vi "prepAO_img.vi"() -> (0 "Terminal Name with Device Prefix":tag)   [LabVIEW 2015]
uses:
  <vilib>/DAQmx/write.llb/DAQmx Write (Analog 1D Wfm NChan NSamp).vi
  waveforms/usedAOindepofwf.vi
  Misc/add channel to active arrayv2.vi
  Objects/waveformsAObuffer.vi
  <vilib>/DAQmx/create/channels.llb/DAQmx Create Channel (AO-Voltage-Basic).vi
  <vilib>/DAQmx/configure/timing.llb/DAQmx Timing (Sample Clock).vi
  <vilib>/DAQmx/miscellaneous.llb/DAQmx Fill In Error Info.vi
  <vilib>/DAQmx/configure/trigger.llb/DAQmx Start Trigger (Digital Edge).vi
panel:
  in  "error in 3":errorcluster caption="error in"
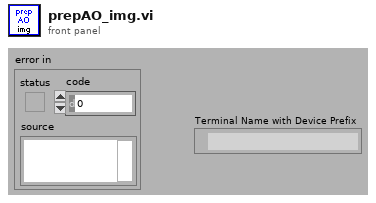
[diagram p1: front panel]
types:
  T1 = cluster{"presorted indices":i32[], "AOchans in this device":tag[], "usedAO sorted":i32[]}[]
  T2 = typedef "LVRectTypeDef.ctl" = cluster{"Left":i16, "Top":i16, "Right":i16, "Bottom":i16}
  T3 = cluster{"Xpixels":i32, "Vxminref":dbl, "Vxmaxref":dbl, "P":dbl, "Ypixels":i32, "Vyminref":dbl, "Vymaxref":dbl, "srate":sgl, "sAOxy":i32, "timeout":dbl, "type":string, "date":string, "time":string, "Colormap":u16, "Drawing Mode":u16, "Scanning Mode":u16, "square pixels":bool, "square matrix":bool, "Xpixels Img":i32, "Vx-min Img":dbl, "VX-max Img":dbl, "Ypixels Img":i32, "Vy-min Img":dbl, "Vy-max Img ":dbl, "Angle Img":dbl, "autoshutter":bool, "finite":bool, "cont":bool, "wavdet":bool, "measpoints":i32, "avpp":i32, "bufferAO":i32, "bufferAI":i32, "starttick":u32, "waveform":path, "Vx-ref":dbl, "Vy-ref":dbl, "refreshrate":dbl, "refreshbuffer":i32, "tt_cycles":i32, "motorref":refnum<k7>, "mirrorswitch":refnum<k7>, "sample mode":i32, "maxbufferAI":i32, "srateAODO":sgl, "bin":sgl, "Pel":sgl, "Angle draw":dbl, "srate Img":sgl, "ROIimg_plotbounds":T2, "auto OD":bool, "ODfilt":u16, "aAI":i32[], "aCI":i32[], "aAO":u32[], "aDO":u32[], "refwfsize":dbl, "Lifetime":bool, "Vz-Img":dbl, "Vz-ref":dbl, "Vz-reset":dbl, "AIoverride":bool}
  T4 = cluster{"StageS":i32, "StageL":i32, "currmeas data dir":path, "image OD":u16, "contour OD":u16, "point OD":u16, "AOlines":tag[], "AIlines":tag[], "CI lines":tag[], "DO lines":tag[], "AO names":string[], "CI names":string[], "AI names":string[], "DO names":string[], "CIextensions":string[], "AIextensions":string[], "Voltage to Ygalvo":i32, "Voltage to Xgalvo":i32, "Voltage to patch":i32, "640 shutter":i32, "2P shutter":i32, "LT timestamp":u32, "Vp":i32, "Ip":i32, "camera trigger":i32, "master data dir":path, "voltage to Zpos":i32, "Vto2P":i32, "640 AO":i32, "488 AO":i32, "532 AO":i32, "640TTL":u32, "488TTL":u32, "532TTL":u32, "Device 1 sampleclock out":tag, "Device 1 Starttrigger out":tag, "Device 2 sampleclock in":tag, "Device 2 StartTrigger in ":tag, "2PODTTL":u32, "488 shutter":u32, "LCVR red":u32, "LCVR blue":u32}
  T5 = cluster{"AO":refnum<k21>[], "E_AO":errorcluster[]}
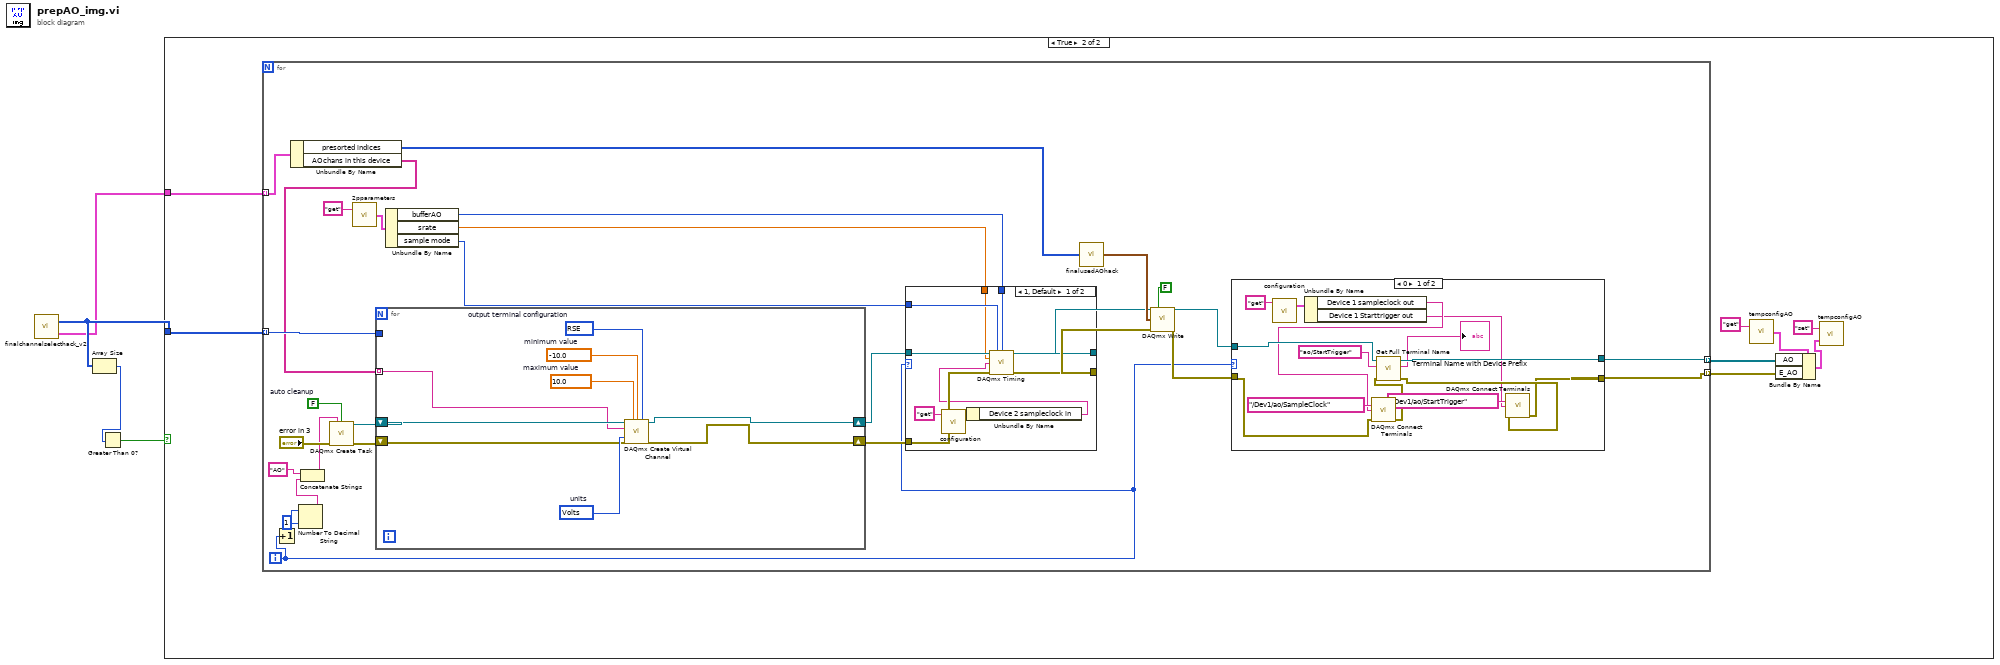
[diagram p0: block diagram]
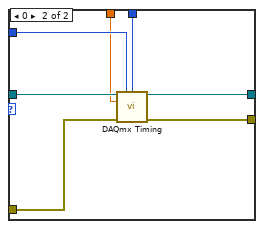
[diagram p3: hidden frame]
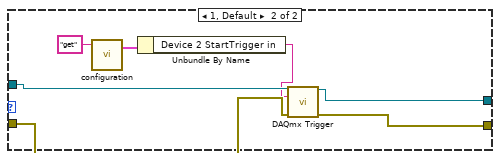
[diagram p4: hidden frame]
diagram:
  n1 = call "finalchannelselecthack_v2.vi"() -> ("devices"=w2:u32[], "Device chans"=w1:T1)  [unwired: 1 in]
  n2 = Array Size(array=w2) -> (size(s)=w3:i32)
  n3 = Greater Than 0?(x=w3) -> (x > 0?=w4:bool)
  n4 = case shown="True" w4 {
    tunnel: w2 -> [_ w5]
    tunnel: w1 -> [_ w12]
    frame False {
    }
    frame True {
      n5 = for {
        tunnel: w5 -> [w37] mode=indexing
        tunnel: w12 -> [w28] mode=indexing
        tunnel: [w15] -> w7 mode=indexing
        tunnel: [w14] -> w6 mode=indexing
        i -> [w13]
        w39 = FALSE  # auto cleanup
        n6 = Increment(x=w13) -> (x+1=w25:i32)
        n7 = Unbundle By Name(w28) -> ("presorted indices"=w21:i32[], "AOchans in this device"=w27:tag[])
        n8 = Number To Decimal String(number=w25, width (-)=i16 1) -> (decimal integer string=w24:string)
        n9 = Concatenate Strings("AO" ("new task name"), w24) -> (w22:string)
        n10 = call <vilib>:"DAQmx Create Task.vi"("new task name"=w22, "auto cleanup"=w39, "error in"="error in 3") -> ("task out"=w40:refnum<k21>, "error out"=w41:errorcluster)  [unwired: 11 in]
        n11 = call "2pparameters.vi"("command"="get") -> ("params out"=w33:T3)  [unwired: 1 in]
        n12 = for {
          shift-right: [w82] -> w36
          shift-left: w40 -> [w84]
          shift-right: [w81] -> w35
          shift-left: w41 -> [w83]
          tunnel: w37 -> [_]
          tunnel: w27 -> [w80] mode=indexing
          w88 = 10083 items=["Default"=-1, "RSE"=10083, "Differential"=10106, "Pseudodifferential"=12529]  # output terminal configuration
          w87 = 10348 items=["Volts"=10348, "From Custom Scale"=10065]  # units
          w86 = -10.0  # minimum value
          w85 = 10.0  # maximum value
          n13 = call-poly <vilib>:"DAQmx Create Virtual Channel.vi"("task in"=w84, "maximum value"=w85, "minimum value"=w86, "output terminal configuration"=w88, "physical channels"=w80, "units"=w87, "error in"=w83) -> ("task out"=w82:refnum<k21>, "error out"=w81:errorcluster)  [unwired: 7 in]
        }
        n14 = Unbundle By Name(w33) -> ("bufferAO"=w30:i32, "srate"=w31:sgl, "sample mode"=w32:i32)
        n15 = case shown="1, Default" w13 {
          tunnel: w36 -> [w51 w58]
          tunnel: w35 -> [w50 w57]
          tunnel: w32 -> [w49 w56]
          tunnel: w31 -> [w48 w55]
          tunnel: w30 -> [w47 w54]
          tunnel: [w46 w53] -> w19
          tunnel: [w45 w52] -> w18
          frame 1, Default {
            n16 = call "configuration.vi"("command"="get") -> ("config out"=w43:T4)  [unwired: 2 in, 1 out]
            n17 = Unbundle By Name(w43) -> ("Device 2 sampleclock in"=w42:tag)
            n18 = call-poly <vilib>:"DAQmx Timing.vi"("task/channels in"=w51, "sample mode"=w49, "samples per channel"=w47, "rate"=w48, "source"=w42, "error in"=w50) -> ("task out"=w45:refnum<k21>, "error out"=w46:errorcluster)  [unwired: 1 in, 7 out]
          }
          frame 0 {
            n19 = call-poly <vilib>:"DAQmx Timing.vi"("task/channels in"=w58, "sample mode"=w56, "samples per channel"=w54, "rate"=w55, "error in"=w57) -> ("task out"=w52:refnum<k21>, "error out"=w53:errorcluster)  [unwired: 2 in, 7 out]
          }
        }
        n20 = call "finalusedAOhack.vi"("presorted indices"=w21) -> ("AO wf out"=w29:waveform(dbl)[])
        n21 = call-poly <vilib>:"DAQmx Write.vi"("task/channels in"=w18, "auto start"=FALSE, "data"=w29, "error in"=w19) -> ("task out"=w17:refnum<k21>, "error out"=w16:errorcluster)  [unwired: 9 in, 1 out]
        n22 = case shown="0" w13 {
          tunnel: [w71 w79] -> w15
          tunnel: [w63 w78] -> w14
          tunnel: w16 -> [w67 w76]
          tunnel: w17 -> [w69 w77]
          frame 0 {
            n23 = call "configuration.vi"("command"="get") -> ("config out"=w62:T4)  [unwired: 2 in, 1 out]
            n24 = Unbundle By Name(w62) -> ("Device 1 sampleclock out"=w60:tag, "Device 1 Starttrigger out"=w59:tag)
            n25 = call <vilib>:"DAQmx Connect Terminals.vi"("source terminal"=tag "/Dev1/ao/SampleClock", "destination terminal"=w60, "error in"=w67) -> ("error out"=w66:errorcluster)  [unwired: 12 in]
            n26 = call "Get Full Terminal Name.vi"("error in"=w66, "Local Terminal Name"="ao/StartTrigger", "task/channels in"=w69) -> ("error out"=w64:errorcluster, "Terminal Name with Device Prefix"=→"Terminal Name with Device Prefix":tag, "task out"=w71:refnum<k21>)  [unwired: 6 in]
            n27 = call <vilib>:"DAQmx Connect Terminals.vi"("source terminal"=tag "/Dev1/ao/StartTrigger", "destination terminal"=w59, "error in"=w64) -> ("error out"=w63:errorcluster)  [unwired: 12 in]
          }
          frame 1, Default {
            n28 = call "configuration.vi"("command"="get") -> ("config out"=w74:T4)  [unwired: 2 in, 1 out]
            n29 = Unbundle By Name(w74) -> ("Device 2 StartTrigger in"=w73:tag)
            n30 = call-poly <vilib>:"DAQmx Trigger.vi"("task/channels in"=w77, "source"=w73, "error in"=w76) -> ("task out"=w79:refnum<k21>, "error out"=w78:errorcluster)  [unwired: 11 in]
          }
        }
      }
      n31 = call "tempconfigAO.vi"("command"="get") -> ("Temp Config out"=w10:T5)  [unwired: 1 in]
      n32 = Bundle By Name(cluster=w10, "AO"=w7, "E_AO"=w6) -> (w11:T5)
      n33 = call "tempconfigAO.vi"("Temp Config in"=w11, "command"="set") -> ()  [unwired: 1 out]
    }
  }
